vi "Get Server State UE.vi"(11 "OOP Query Server in":refnum<class "OOP Query Server.lvclass">) -> (2 "Server Internal State UE":refnum<user-event>, 3 "OOP Query Server out":refnum<class "OOP Query Server.lvclass">)   [LabVIEW 2019, in "OOP Query Server.lvlib" / "OOP Query Server.lvclass"]
uses:
  OOP Query Server.lvclass
  typeDefs/Server State Data.ctl
  OOP Query Server.lvclass/OOP Query Server.ctl
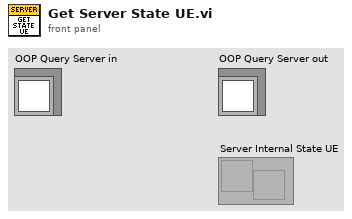
[diagram p1: front panel]
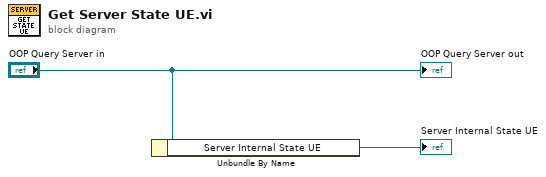
[diagram p0: block diagram]
diagram:
  n1 = Unbundle By Name("OOP Query Server in") -> ("Server Internal State UE"=→"Server Internal State UE":refnum<user-event>)
  "OOP Query Server out" <- "OOP Query Server in"
